vi "Write Roles.vi"(8 "error in (no error)":errorcluster, 10 "Roles":T1, 11 "GoalKickEnemyPlayVSS in":refnum<class "GoalKickEnemyPlayVSS.lvclass">) -> (0 "error out":errorcluster, 3 "GoalKickEnemyPlayVSS out":refnum<class "GoalKickEnemyPlayVSS.lvclass">)   [LabVIEW 2023, in "GoalKickEnemyPlayVSS.lvclass"]
uses:
  GoalKickEnemyPlayVSS.lvclass
  KeeperRoleVSS_class/KeeperRoleVSS.lvclass
  DefenderAreaRoleVSS_class/DefenderAreaRoleVSS.lvclass
  HaltRole_class/HaltRole.lvclass
  GoalKickEnemyPlayVSS.lvclass/GoalKickEnemyPlayVSS.ctl
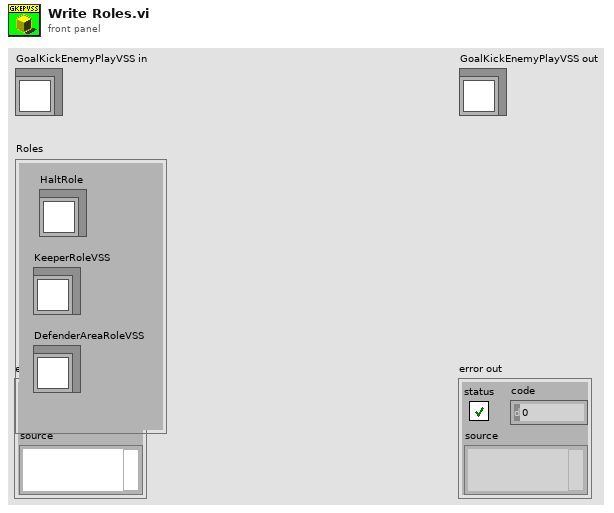
[diagram p1: front panel]
types:
  T1 = cluster{"KeeperRoleVSS":refnum<class "KeeperRoleVSS.lvclass">, "DefenderAreaRoleVSS":refnum<class "DefenderAreaRoleVSS.lvclass">, "HaltRole":refnum<class "HaltRole.lvclass">}
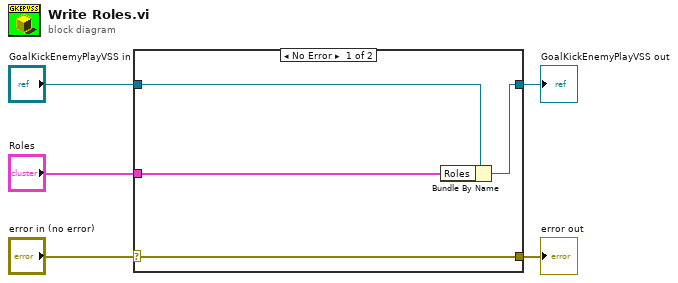
[diagram p0: block diagram]
diagram:
  n1 = case shown="No Error" "error in (no error)" {
    selector: "error in (no error)" -> [w9 w10]
    tunnel: [w9 w10] -> w4
    tunnel: [w7 w11] -> w2
    tunnel: "GoalKickEnemyPlayVSS in" -> [w8 w11]
    tunnel: "Roles" -> [w6 _]
    frame No Error {
      n2 = Bundle By Name(cluster=w8, "Roles"=w6) -> (w7:refnum<class "GoalKickEnemyPlayVSS.lvclass">)
    }
    frame Error {
    }
  }
  "error out" <- w4
  "GoalKickEnemyPlayVSS out" <- w2
